vi "TopPortV2.vi"(8 "error in (no error)":errorcluster, 11 "Image Src":T1) -> (0 "error out":errorcluster, 2 "Shape Report":T2(array[cluster]) {"Score" format="%.2f"; "Centroid"."y" format="%.2f"; "Centroid"."x" format="%.2f"}, 3 "Number of Matches":i32)   [LabVIEW 2019]
uses:
  <vilib>/vision/Image Controls.llb/IMAQ Image.ctl
  <vilib>/vision/NI_Vision_Development_Module.lvlib
panel:
  out "x*y":sgl
  out "Mean Value":sgl
  in  "y":sgl
  in  "Minimal Score":dbl=2.0 format="%.2f"
  out "Image Out":T1(plugin-control)
  out "Histogram (Histogram 1)":u32[][](array[numeric])
  out "Histogram Graph":u32[][](graph)
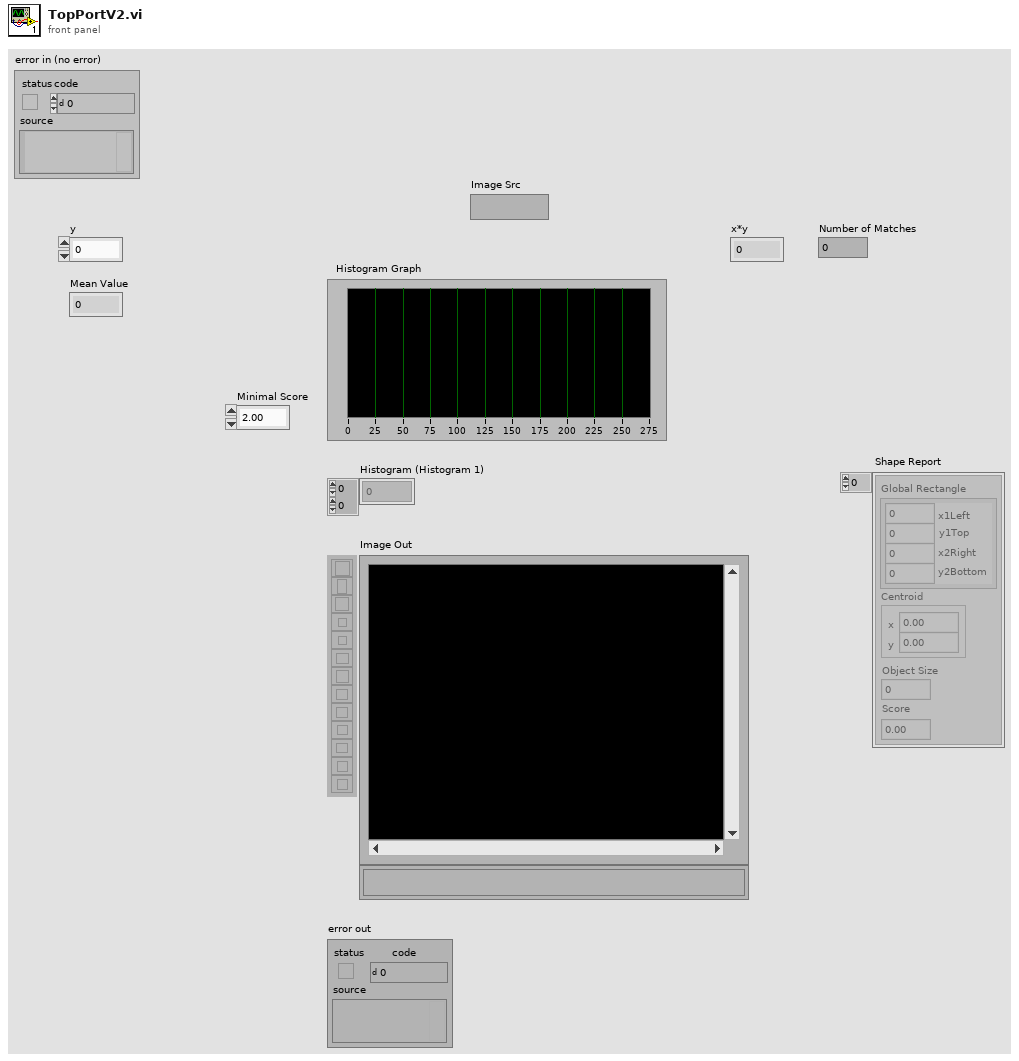
[diagram p1: front panel]
types:
  T1 = typedef "IMAQ Image.ctl" = refnum<image>
  T2 = cluster{"Global Rectangle":cluster{"x1Left":i32, "y1Top":i32, "x2Right":i32, "y2Bottom":i32}, "Centroid":cluster{"x":sgl, "y":sgl}, "Object Size":u32, "Score":dbl}[]
  T3 = cluster{"Measurement Parameter":i32, "Range Lower Value":dbl, "Range Upper Value":dbl, "Range":bool, "Measurement Type":bool}[]
  T4 = enum32{"AutoM", "Close", "Dilate", "Erode", "Gradient", "Gradient in", "Gradient out", "HitMiss", "Open", "PClose", "POpen", "Thick", "Thin"}
  T5 = cluster{"Global Rectangle":i32[], "Contours":cluster{"ID":enum32{"External", "Internal"}, "Type":u32, "Coordinates":i32[]}[]}
  T6 = cluster{"Minimal Value":sgl, "Maximal Value":sgl, "Mean Value":sgl, "Standard  Variation":sgl, "Area (pixels)":i32}
  T7 = cluster{"histogram":u32[], "Minimal Value":sgl, "Maximal Value":sgl, "Starting Value":sgl, "Interval Width":sgl, "Mean Value":sgl, "Standard  Variation":sgl, "Area (pixels)":i32}
  T8 = typedef "Image Type" = u32
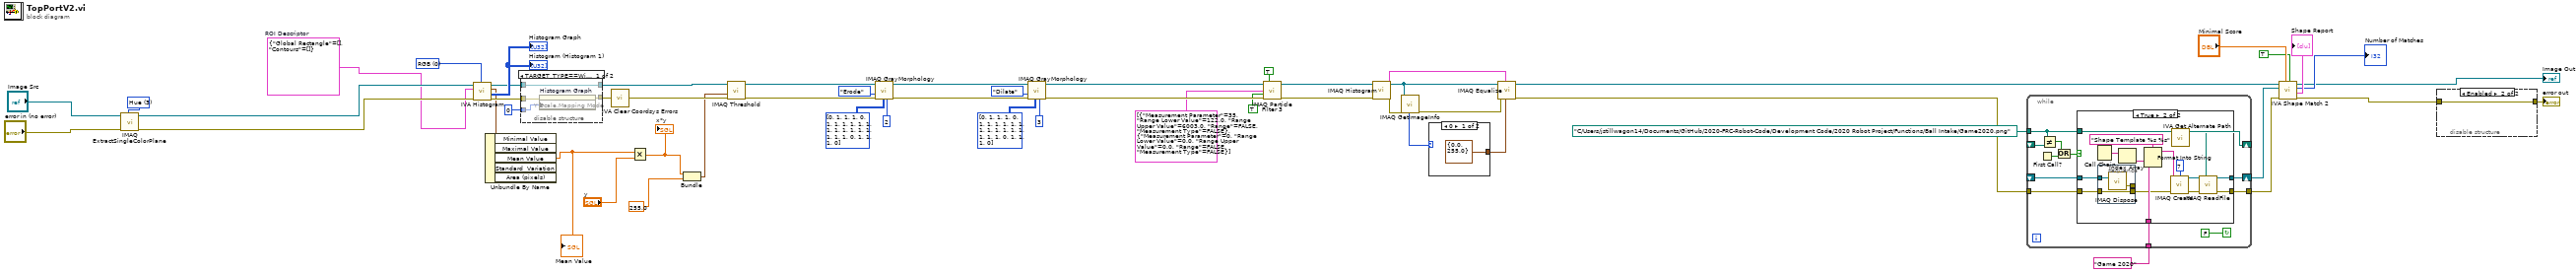
[diagram p0: block diagram]
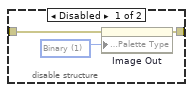
[diagram p2: hidden frame]
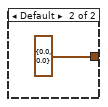
[diagram p4: hidden frame]
diagram:
  w51 = u16 0 items=["RGB", "HSL", "HSV", "HSI"] ("Color Mode")
  w49 = T5 {"Global Rectangle"=[], "Contours"=[]}  # ROI Descriptor
  w55 = 3 items=["Red", "Green", "Blue", "Hue", "Saturation", "Luminance", "Value", "Intensity"] ("Color Plane")
  n1 = call "IMAQ ExtractSingleColorPlane"("Color Plane"=w55, "error in (no error)"="error in (no error)", "Image Src"="Image Src") -> ("error out"=w54:errorcluster, "Image Dst Out"=w53:T1)  [unwired: 1 in, 6 out]
  n2 = call <vilib>:"IVA Histogram.vi"("Color Mode"=w51, "error in (no error)"=w54, "ROI Descriptor"=w49, "Image In"=w53) -> ("error out"=w52:errorcluster, "Histograms"=→"Histogram Graph" →"Histogram (Histogram 1)":u32[][], "Statistics"=w11:T6, "Image Out"=w48:T1)  [unwired: 4 out]
  n3 = Unbundle By Name(w11) -> ("Mean Value"=w9:sgl)  [unwired: 4 out]
  "Mean Value" <- w9
  n4 = disable-structure "Conditional Disable Structure" shown="TARGET_TYPE==Windows" {
    disable-tunnel: w52 -> [w59 w60]
    disable-tunnel: [w58 w60] -> w46
    disable-tunnel: w48 -> [w57 w61]
    disable-tunnel: [w57 w61] -> w44
    disable-tunnel: u8 0 ("Y Scale.Mapping Mode") -> [w56 _]
    frame condition #0 {
      n5 = property on="Histogram Graph" class="WFGraph (strict)"(error in=w59, "Y Scale.Mapping Mode"=w56) -> (error out=w58:errorcluster)  [unwired: 1 in, 1 out]
    }
    frame condition #1 (active) {
    }
  }
  n6 = call <vilib>:"IVA Clear Coordsys Errors.vi"("error in (no error)"=w46) -> ("error out"=w45:errorcluster)  [unwired: 10 in]
  n7 = Multiply(x=w9, y="y") -> (x*y=w7:sgl)
  "x*y" <- w7
  n8 = Bundle(w7, "Upper value"=sgl 255.0) -> (w6:cluster{sgl, "Upper value":sgl})  [unwired: 1 in]
  n9 = call "IMAQ Threshold"("error in (no error)"=w45, "Range"=w6, "Image Src"=w44) -> ("error out"=w43:errorcluster, "Image Dst Out"=w40:T1)  [unwired: 3 in, 4 out]
  n10 = call "IMAQ GrayMorphology"("Number of iterations (1)"=2, "Structuring Element"=i32[][] [[0, 1, 1, 1, 0], [1, 1, 1, 1, 1], [1, 1, 1, 1, 1], [1, 1, 1, 1, 1], [0, 1, 1, 1, 0]], "error in (no error)"=w43, "Operation"=T4."Erode", "Image Src"=w40) -> ("error out"=w39:errorcluster, "Image Dst Out"=w35:T1)  [unwired: 2 in, 3 out]
  n11 = call "IMAQ GrayMorphology"("Number of iterations (1)"=3, "Structuring Element"=i32[][] [[0, 1, 1, 1, 0], [1, 1, 1, 1, 1], [1, 1, 1, 1, 1], [1, 1, 1, 1, 1], [0, 1, 1, 1, 0]], "error in (no error)"=w39, "Operation"=T4."Dilate", "Image Src"=w35) -> ("error out"=w34:errorcluster, "Image Dst Out"=w29:T1)  [unwired: 2 in, 3 out]
  n12 = call "IMAQ Particle Filter 3"("Image Src"=w29, "Connectivity 4/8 (8)"=TRUE, "Selection Values"=T3 [{"Measurement Parameter"=35, "Range Lower Value"=122.0, "Range Upper Value"=6003.0, "Range"=FALSE, "Measurement Type"=FALSE}, {"Measurement Parameter"=0, "Range Lower Value"=0.0, "Range Upper Value"=0.0, "Range"=FALSE, "Measurement Type"=FALSE}], "Keep/Remove Particles (F)"=TRUE ("Keep/Remove Particles"), "error in (no error)"=w34) -> ("Image Dst Out"=w24:T1, "error out"=w30:errorcluster)  [unwired: 4 in, 5 out]
  n13 = call "IMAQ Histogram"("error in (no error)"=w30, "Image"=w24) -> ("error out"=w23:errorcluster, "Histogram Report"=w26:T7)  [unwired: 3 in, 5 out]
  n14 = call "IMAQ GetImageInfo"("error in (no error)"=w23, "Image"=w24) -> ("error out"=w22:errorcluster, "Image Type"=w25:T8)  [unwired: 8 out]
  n15 = case shown="0" w25 {
    tunnel: [cluster{"Minimum":sgl, "Maximum":sgl} {"Minimum"=0.0, "Maximum"=255.0} ("Range") cluster{"Minimum":sgl, "Maximum":sgl} {"Minimum"=0.0, "Maximum"=0.0} ("Range")] -> w21
    frame 0 {
    }
    frame Default {
    }
  }
  n16 = call "IMAQ Equalize"("Range"=w21, "Histogram Report"=w26, "error in (no error)"=w22, "Image Src"=w24) -> ("error out"=w27:errorcluster, "Image Dst Out"=w18:T1)  [unwired: 2 in, 4 out]
  n17 = while {
    shift-right: [w74] -> w14
    shift-left: _ -> [w73]
    tunnel: [w71] -> w15
    tunnel: w27 -> [w70]
    tunnel: path "C:/Users/jstillwagon14/Documents/GitHub/2020-FRC-Robot-Code/Development Code/2020 Robot Project/Functions/Ball Intake/Game2020.png" ("Template Path") -> [w68]
    tunnel: "Game 2020" ("Step Name") -> [w69]
    shift-right: [w68] -> _
    shift-left: _ -> [w67]
    stop <- FALSE continue-if-true
    n18 = First Call?() -> (First Call?: T/F=w66:bool)
    n19 = Not Equal?(x=w68, y=w67) -> (x != y?=w65:bool)
    n20 = Or(x=w65, y=w66) -> (x .or. y?=w64:bool)
    n21 = case shown="True" w64 {
      tunnel: [w76 w88] -> w74
      tunnel: w73 -> [w76 w79]
      tunnel: [w75 w86] -> w71
      tunnel: w70 -> [w75 w78]
      tunnel: w68 -> [_ w81]
      tunnel: w69 -> [_ w82]
      frame False {
      }
      frame True {
        n22 = Call Chain() -> (call chain=w84:string[])
        n23 = stacked-sequence {
          tunnel: w79 -> [w94]
          tunnel: w78 -> [w93]
          tunnel: [w93] -> w77
          tunnel: [w92] -> _
          frame #0 {
            n24 = call "IMAQ Dispose"("Image"=w94) -> ("error out"=w92:errorcluster)  [unwired: 2 in, 3 out]
          }
        }
        n25 = Index Array(array=w84) -> (element=w83:string)  [unwired: 1 in]
        n26 = Format Into String(format string="Shape Template %s %s" ("Image Name"), w83, w82) -> (resulting string=w91:string)  [unwired: 2 in, 1 out]
        n27 = call "IMAQ Create"("Border Size"=7, "Image Name"=w91, "error in (no error)"=w77) -> ("New Image"=w89:T1, "error out"=w87:errorcluster)  [unwired: 1 in, 1 out]
        n28 = call <vilib>:"IVA Get Alternate Path.vi"("Path In"=w81) -> ("Path Out"=w80:path)  [unwired: 10 out]
        n29 = call "IMAQ ReadFile"("File Path"=w80, "error in (no error)"=w87, "Image"=w89) -> ("error out"=w86:errorcluster, "Image Out"=w88:T1)  [unwired: 2 in, 5 out]
      }
    }
  }
  n30 = call <vilib>:"IVA Shape Match 2.vi"("Scale Invariance"=TRUE, "Minimal Score"="Minimal Score", "error in (no error)"=w15, "Template"=w14, "Image Src"=w18) -> ("error out"=w1:errorcluster, "Shape Report"=→"Shape Report":T2, "Number of Matches"=→"Number of Matches":i32, "Image Out"=→"Image Out":T1)  [unwired: 3 out]
  n31 = disable-structure shown="Enabled" {
    disable-tunnel: w1 -> [w97 w98]
    disable-tunnel: [w96 w98] -> w12
    frame Disabled {
      w95 = u32 1 items=["Grayscale", "Binary", "Gradient", "Rainbow", "Temperature", "User Defined", "Binary 16 Bit", "Gradient 16 Bit", "Rainbow 16 Bit", "Temperature 16 Bit", "User Defined 16 Bit"] ("Palette Type")
      n32 = property on="Image Out" class="ImageControl"(error in=w97, "Palette:Palette Type"=w95) -> (error out=w96:errorcluster)  [unwired: 1 in, 1 out]
    }
    frame Enabled {
    }
  }
  "error out" <- w12
